vi "Destroy.vi"(8 "Error In":errorcluster, 11 "reference in":refnum<class "Circle.lvclass">) -> (0 "Error Out":errorcluster, 3 "reference out":refnum<class "Circle.lvclass">)   [LabVIEW 2020, in "Circle.lvclass"]
uses:
  Circle.lvclass
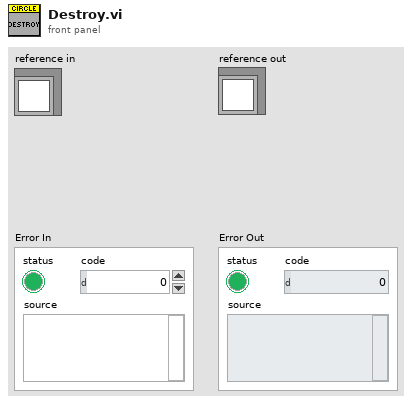
[diagram p1: front panel]
types:
  T1 = typedef "Circle.lvclass/ObjectAttributes.ctl" = cluster{"_radius":i32}
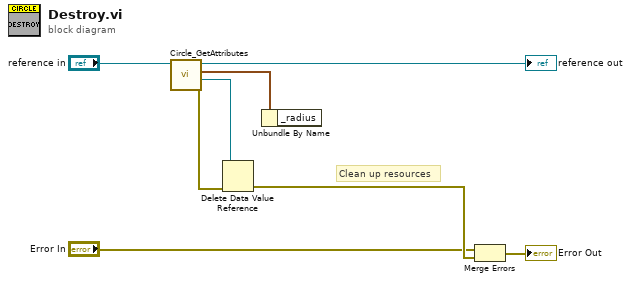
[diagram p0: block diagram]
diagram:
  # "Clean up resources"
  n1 = call "Circle_GetAttributes.vi"("reference in"="reference in") -> ("error out"=w5:errorcluster, "DataRef"=w4:refnum<data-value>, "Data"=w3:T1, "reference out"=→"reference out":refnum<class "Circle.lvclass">)  [unwired: 7 in]
  n2 = Delete Data Value Reference(data value reference=w4, error in=w5) -> (error out=w2:errorcluster)  [unwired: 1 out]
  n3 = Unbundle By Name(w3) -> ()  [unwired: 1 out]
  n4 = Merge Errors("Error In", w2) -> (→"Error Out":errorcluster)
